vi "Generate Bursted Script.vi"(0 "PAEN Config":T1={"PAEN Mode"=enum."Dynamic", "PA Enable Trigger Export Terminal"="PFI0", "PA Enable Trigger Mode"=23001, "Command Enable Time (s)"=0.0, "Command Disable Time (s)"=0.0} {"PA Enable Trigger Mode" items=["Pulse"=23000, "Toggle"=23001]; "Command Disable Time (s)" format="%#_6p"; "Command Enable Time (s)" format="%#_6p"}, 5 "Waveform Timing Configuration":T4 {"Post-Burst Time (s)" format="%#_6p"; "Pre-Burst Time (s)" format="%#_6p"; "Duty Cycle (%)" min=1.0 max=100.0 step=1.0 format="%#_2d%%"}, 7 "Waveform":T3 {"Runtime Scaling" format="%#_6p"; "Sample Rate" format="%#_6p"; "Burst Length (s)" format="%#_6p"; "PAPR (dB)" format="%.2f"; "Signal Bandwidth (Hz)" format="%#_6p"}, 11 "error in (no error)":errorcluster) -> (4 "Script":string, 6 "Generation Period (s)":dbl, 15 "error out":errorcluster)   [LabVIEW 2019, in "SG.lvlib"]
doc: "Creates the generation script used for bursted generation."
uses:
  SG.lvlib
  Typedefs/Waveform Timing Configuration.ctl
  <instrlib>/niRFSG/niRFSG.llb/niRFSG Exported Signal Destinations.ctl
  Common/Waveform.ctl
  Typedefs/PAEN Configuration.ctl
  <vilib>/Utility/error.llb/Error Cluster From Error Code.vi
  <vilib>/ErrorRing/Error Ring.xnode
  Common/Common.lvlib
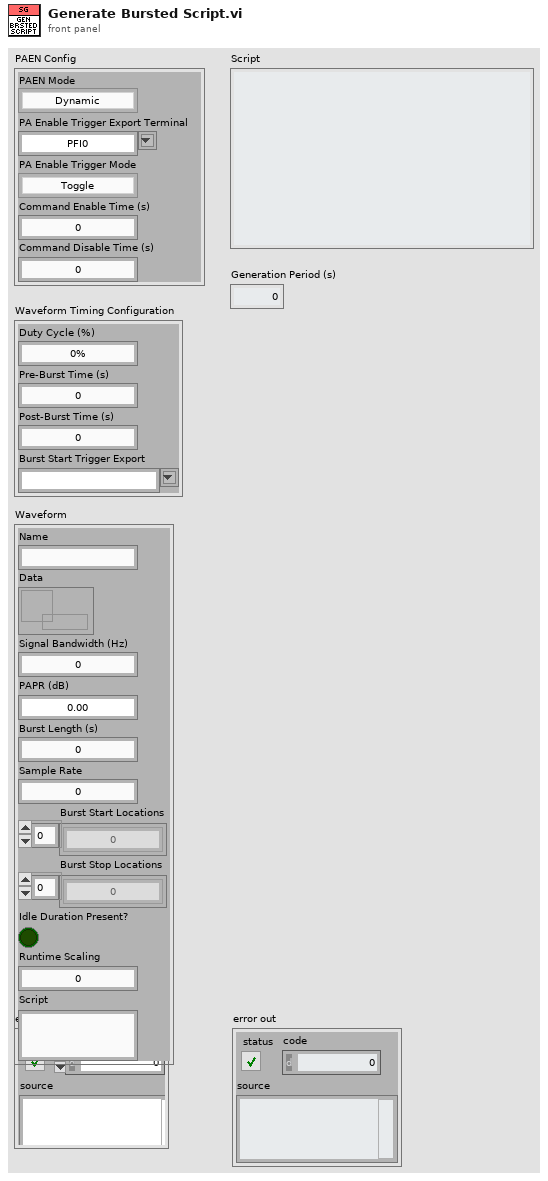
[diagram p1: front panel]
types:
  T1 = typedef "SG.lvlib/PAEN Configuration.ctl" = cluster{"PAEN Mode":enum16{"Disabled", "Static", "Dynamic"}, "PA Enable Trigger Export Terminal":T2, "PA Enable Trigger Mode":i32, "Command Enable Time (s)":dbl, "Command Disable Time (s)":dbl}
  T2 = typedef "niRFSG Exported Signal Destinations.ctl" = string
  T3 = typedef "Common.lvlib/Waveform.ctl" = cluster{"Name":string, "Data":refnum<data-value>, "Signal Bandwidth (Hz)":dbl, "PAPR (dB)":dbl, "Burst Length (s)":dbl, "Sample Rate":dbl, "Burst Start Locations":i32[], "Burst Stop Locations":i32[], "Idle Duration Present?":bool, "Runtime Scaling":dbl, "Script":string}
  T4 = typedef "SG.lvlib/Waveform Timing Configuration.ctl" = cluster{"Duty Cycle (%)":dbl, "Pre-Burst Time (s)":dbl, "Post-Burst Time (s)":dbl, "Burst Start Trigger Export":T2}
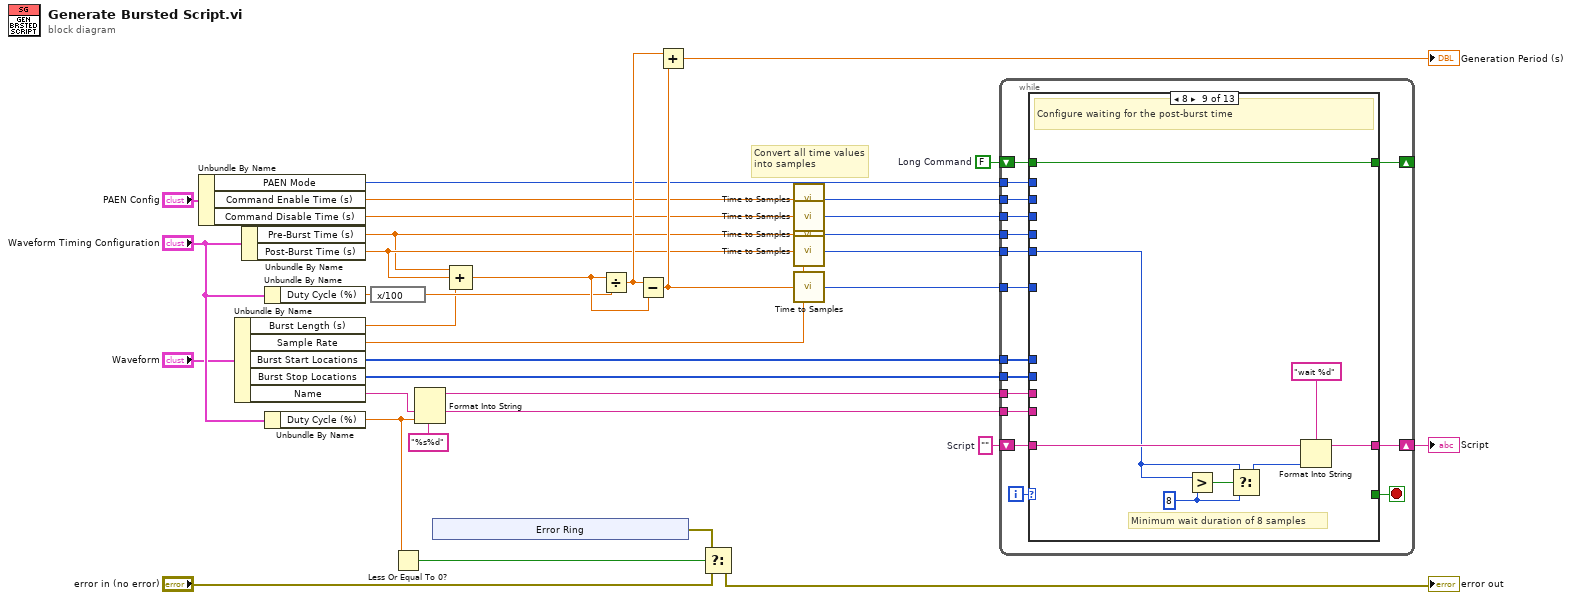
[diagram p0: block diagram]
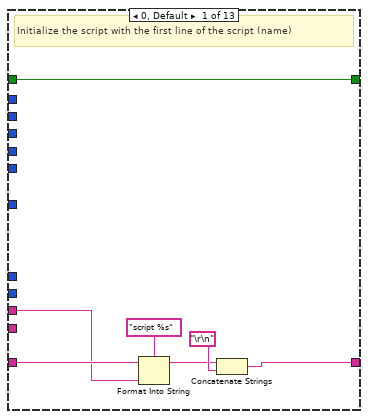
[diagram p2: hidden frame]
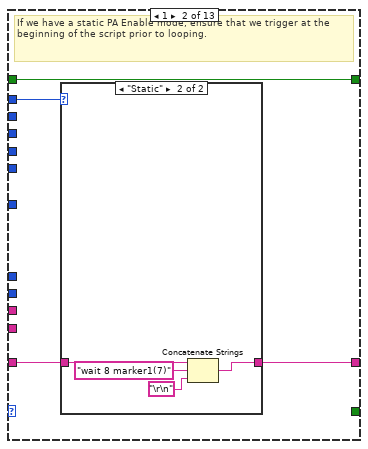
[diagram p3: hidden frame]
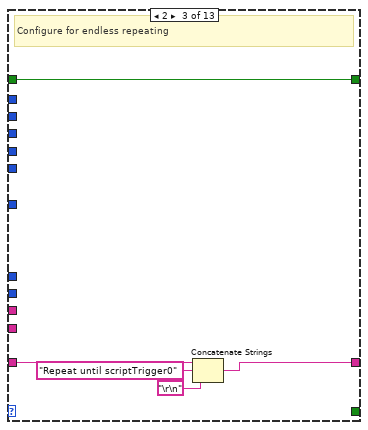
[diagram p5: hidden frame]
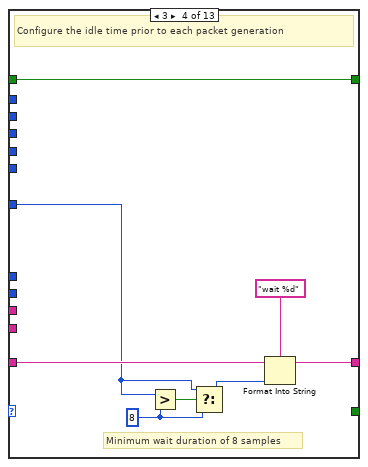
[diagram p6: hidden frame]
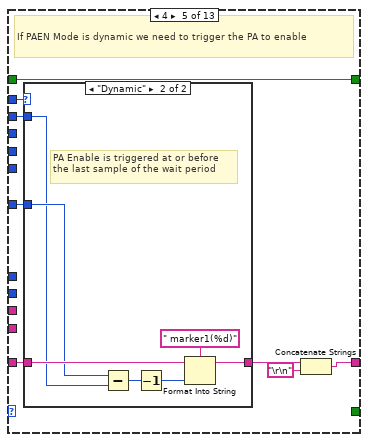
[diagram p7: hidden frame]
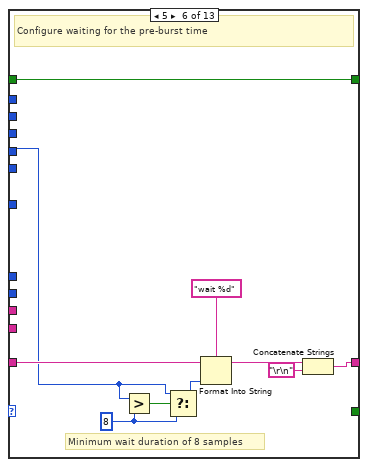
[diagram p9: hidden frame]
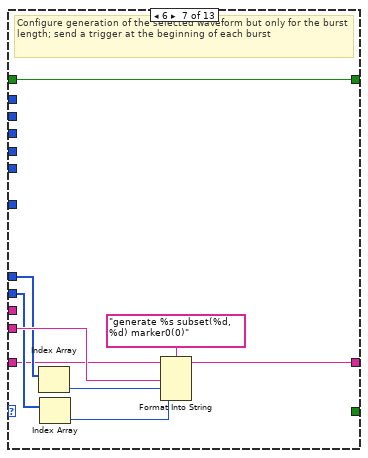
[diagram p10: hidden frame]
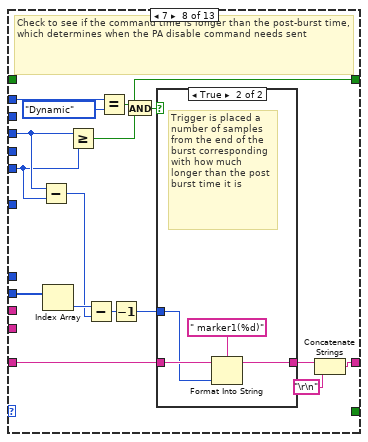
[diagram p11: hidden frame]
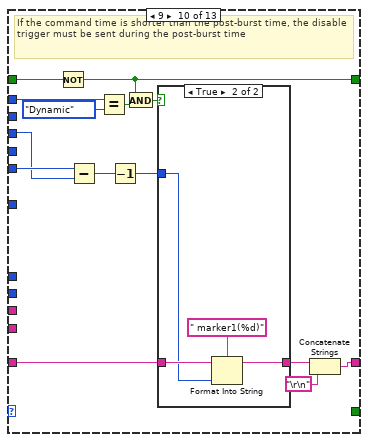
[diagram p13: hidden frame]
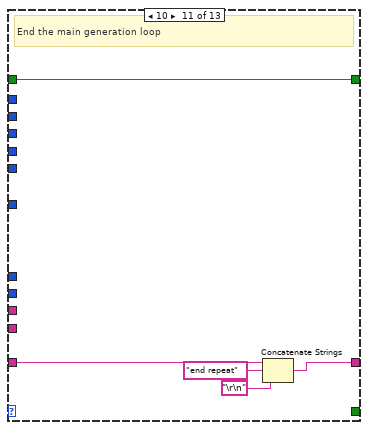
[diagram p15: hidden frame]
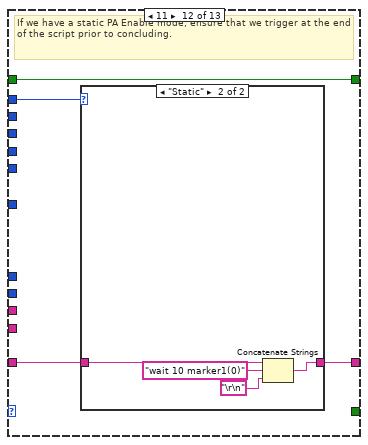
[diagram p16: hidden frame]
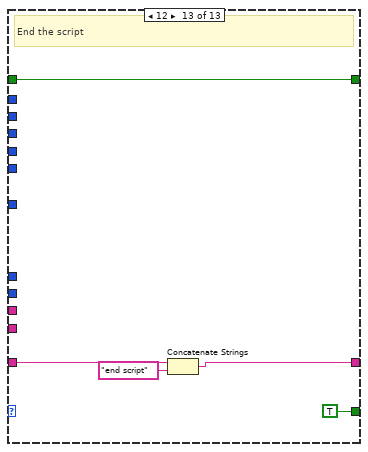
[diagram p18: hidden frame]
diagram:
  w30 = FALSE  # Long Command
  w25 = ""  # Script
  # "Convert all time values into samples"
  n1 = Unbundle By Name("PAEN Config") -> ("PAEN Mode"=w26:enum16{"Disabled", "Static", "Dynamic"}, "Command Enable Time (s)"=w9:dbl, "Command Disable Time (s)"=w10:dbl)
  n2 = Unbundle By Name("Waveform") -> ("Burst Length (s)"=w13:dbl, "Sample Rate"=w18:dbl, "Burst Start Locations"=w28:i32[], "Burst Stop Locations"=w29:i32[], "Name"=w27:string)
  n3 = Unbundle By Name("Waveform Timing Configuration") -> ("Pre-Burst Time (s)"=w11:dbl, "Post-Burst Time (s)"=w12:dbl)
  n4 = Unbundle By Name("Waveform Timing Configuration") -> ("Duty Cycle (%)"=w15:dbl)
  n5 = Unbundle By Name("Waveform Timing Configuration") -> ("Duty Cycle (%)"=w32:dbl)
  n6 = expression code="x/100"(w15) -> (w16:dbl)
  n7 = Less Or Equal To 0?(x=w32) -> (x <= 0?=w6:bool)
  n8 = Format Into String(format string="%s%d", w27, w32) -> (resulting string=w24:string)  [unwired: 2 in, 1 out]
  n9 = xnode "Error Ring"() -> ("error out"=w1:errorcluster)
  n10 = Compound Arithmetic op=ADD(w11, w12, w13) -> (w17:dbl)
  n11 = Divide(x=w17, y=w16) -> (x/y=w33:dbl)
  n12 = Subtract(x=w33, y=w17) -> (x-y=w34:dbl)
  n13 = Add(x=w33, y=w34) -> (x+y=→"Generation Period (s)":dbl)
  n14 = Select(t=w1, s=w6, f="error in (no error)") -> (s? t:f=→"error out":errorcluster)
  n15 = call "Time to Samples.vi"("Time"=w9, "Sample Rate"=w18) -> ("Samples"=w19:u32)  [unwired: 13 in]
  n16 = call "Time to Samples.vi"("Time"=w10, "Sample Rate"=w18) -> ("Samples"=w20:u32)  [unwired: 13 in]
  n17 = call "Time to Samples.vi"("Time"=w11, "Sample Rate"=w18) -> ("Samples"=w21:u32)  [unwired: 13 in]
  n18 = call "Time to Samples.vi"("Time"=w12, "Sample Rate"=w18) -> ("Samples"=w22:u32)  [unwired: 13 in]
  n19 = call "Time to Samples.vi"("Time"=w34, "Sample Rate"=w18) -> ("Samples"=w23:u32)  [unwired: 13 in]
  n20 = while {
    tunnel: w19 -> [w43]
    tunnel: w20 -> [w38]
    tunnel: w21 -> [w45]
    tunnel: w22 -> [w39]
    tunnel: w23 -> [w44]
    tunnel: w24 -> [w48]
    shift-right: [w47] -> w31
    shift-left: w25 -> [w49]
    tunnel: w26 -> [w46]
    tunnel: w27 -> [w42]
    tunnel: w28 -> [w41]
    tunnel: w29 -> [w40]
    shift-right: [w37] -> _
    shift-left: w30 -> [w36]
    i -> [w50]
    stop <- w35 stop-if-true
    n21 = case shown="8" w50 {
      tunnel: w49 -> [w57 w60 w71 w79 w87 w105 w109 w127 w143 w154 w165 w171 w180]
      tunnel: w48 -> [w55 _ _ _ _ _ _ _ _ _ _ _ _]
      tunnel: [w52 w59 w70 w77 w81 w101 w113 w120 w141 w151 w167 w170 w179] -> w47
      tunnel: w46 -> [_ w61 _ _ w86 _ _ w130 _ w157 _ w168 _]
      tunnel: w45 -> [_ _ _ _ _ w96 _ _ _ _ _ _ _]
      tunnel: w44 -> [_ _ _ w75 w84 _ _ _ _ _ _ _ _]
      tunnel: w43 -> [_ _ _ _ w85 _ _ _ _ _ _ _ _]
      tunnel: w42 -> [_ _ _ _ _ _ w112 _ _ _ _ _ _]
      tunnel: w41 -> [_ _ _ _ _ _ w111 _ _ _ _ _ _]
      tunnel: w40 -> [_ _ _ _ _ _ w110 w124 _ _ _ _ _]
      tunnel: w39 -> [_ _ _ _ _ _ _ w117 w136 w148 _ _ _]
      tunnel: w38 -> [_ _ _ _ _ _ _ w118 _ w147 _ _ _]
      tunnel: [w51 w58 w67 w76 w80 w100 w106 w115 w140 w144 w166 w169 w181] -> w37
      tunnel: w36 -> [w51 w58 w67 w76 w80 w100 w106 _ w140 w149 w166 w169 w181]
      tunnel: [_ _ _ _ _ _ _ _ _ _ _ _ TRUE] -> w35
      frame 0, Default {
        # "Initialize the script with the first line of the script (name)"
        n22 = Format Into String(format string="script %s", initial string=w57, w55) -> (resulting string=w53:string)  [unwired: 1 in, 1 out]
        n23 = Concatenate Strings(w53, "\r\n") -> (w52:string)
      }
      frame 1 {
        # "If we have a static PA Enable mode, ensure that we trigger at the beginning of the script prior to looping."
        n24 = case shown="\"Static\"" w61 {
          tunnel: w60 -> [w62 w66]
          tunnel: [w62 w65] -> w59
          frame Default {
          }
          frame "Static" {
            n25 = Concatenate Strings(w66, "wait 8 marker1(7)", "\r\n") -> (w65:string)
          }
        }
      }
      frame 2 {
        # "Configure for endless repeating"
        n26 = Concatenate Strings(w71, "Repeat until scriptTrigger0" ("string"), "\r\n" ("string")) -> (w70:string)
      }
      frame 3 {
        w73 = u32 8 ("y")
        # "Minimum wait duration of 8 samples"
        # "Configure the idle time prior to each packet generation"
        n27 = Greater?(x=w75, y=w73) -> (0:w74:bool)
        n28 = Select(t=w75, s=w74, f=w73) -> (s? t:f=w72:u32)
        n29 = Format Into String(format string="wait %d", initial string=w79, w72) -> (resulting string=w77:string)  [unwired: 1 in, 1 out]
      }
      frame 4 {
        # "If PAEN Mode is dynamic we need to trigger the PA to enable"
        n30 = case shown="\"Dynamic\"" w86 {
          tunnel: w87 -> [w88 w95]
          tunnel: [w88 w93] -> w82
          tunnel: w85 -> [_ w91]
          tunnel: w84 -> [_ w92]
          frame Default {
          }
          frame "Dynamic" {
            # "PA Enable is triggered at or before the last sample of the wait period"
            n31 = Subtract(x=w92, y=w91) -> (x-y=w90:u32)
            n32 = Decrement(x=w90) -> (x-1=w89:u32)
            n33 = Format Into String(format string=" marker1(%d)", initial string=w95, w89) -> (resulting string=w93:string)  [unwired: 1 in, 1 out]
          }
        }
        n34 = Concatenate Strings(w82, "\r\n" ("string")) -> (w81:string)
      }
      frame 5 {
        w98 = u32 8 ("y")
        # "Minimum wait duration of 8 samples"
        # "Configure waiting for the pre-burst time"
        n35 = Greater?(x=w96, y=w98) -> (0:w99:bool)
        n36 = Select(t=w96, s=w99, f=w98) -> (s? t:f=w97:u32)
        n37 = Format Into String(format string="wait %d", initial string=w105, w97) -> (resulting string=w102:string)  [unwired: 1 in, 1 out]
        n38 = Concatenate Strings(w102, "\r\n" ("string")) -> (w101:string)
      }
      frame 6 {
        # "Configure generation of the selected waveform but only for the burst length; send a trigger at the beginning of each burst"
        n39 = Index Array(array=w111) -> (element=w108:i32)  [unwired: 1 in]
        n40 = Index Array(array=w110) -> (element=w107:i32)  [unwired: 1 in]
        n41 = Format Into String(format string="generate %s subset(%d, %d) marker0(0)", initial string=w109, w112, w108, w107) -> (resulting string=w113:string)  [unwired: 1 in, 1 out]
      }
      frame 7 {
        # "Check to see if the command time is longer than the post-burst time, which determines when the PA disable command needs sent"
        n42 = Subtract(x=w118, y=w117) -> (x-y=w122:u32)
        n43 = Index Array(array=w124) -> (element=w123:i32)  [unwired: 1 in]
        n44 = Greater Or Equal?(x=w118, y=w117) -> (x >= y?=w115:bool)
        n45 = Subtract(x=w123, y=w122) -> (x-y=w121:u32)
        n46 = Equal?(x=w130, y=enum16{"Disabled", "Static", "Dynamic"}."Dynamic") -> (x = y?=w128:bool)
        n47 = Decrement(x=w121) -> (x-1=w116:u32)
        n48 = And(x=w128, y=w115) -> (x .and. y?=w125:bool)
        n49 = case shown="True" w125 {
          tunnel: w127 -> [w131 w135]
          tunnel: [w131 w134] -> w126
          tunnel: w116 -> [_ w132]
          frame False {
          }
          frame True {
            # "Trigger is placed a number of samples from the end of the burst corresponding with how much longer than the post burst time it is"
            n50 = Format Into String(format string=" marker1(%d)", initial string=w135, w132) -> (resulting string=w134:string)  [unwired: 1 in, 1 out]
          }
        }
        n51 = Concatenate Strings(w126, "\r\n" ("string")) -> (w120:string)
      }
      frame 8 {
        w138 = u32 8 ("y")
        # "Minimum wait duration of 8 samples"
        # "Configure waiting for the post-burst time"
        n52 = Greater?(x=w136, y=w138) -> (0:w139:bool)
        n53 = Select(t=w136, s=w139, f=w138) -> (s? t:f=w137:u32)
        n54 = Format Into String(format string="wait %d", initial string=w143, w137) -> (resulting string=w141:string)  [unwired: 1 in, 1 out]
      }
      frame 9 {
        # "If the command time is shorter than the post-burst time, the disable trigger must be sent during the post-burst time"
        n55 = Not(x=w149) -> (.not. x?=w144:bool)
        n56 = Subtract(x=w148, y=w147) -> (x-y=w146:u32)
        n57 = Equal?(x=w157, y=enum16{"Disabled", "Static", "Dynamic"}."Dynamic") -> (x = y?=w155:bool)
        n58 = Decrement(x=w146) -> (x-1=w145:u32)
        n59 = And(x=w144, y=w155) -> (x .and. y?=w152:bool)
        n60 = case shown="True" w152 {
          tunnel: w154 -> [w158 w162]
          tunnel: [w158 w161] -> w153
          tunnel: w145 -> [_ w159]
          frame False {
          }
          frame True {
            n61 = Format Into String(format string=" marker1(%d)", initial string=w162, w159) -> (resulting string=w161:string)  [unwired: 1 in, 1 out]
          }
        }
        n62 = Concatenate Strings(w153, "\r\n" ("string")) -> (w151:string)
      }
      frame 10 {
        # "End the main generation loop"
        n63 = Concatenate Strings(w165, "end repeat" ("format string"), "\r\n" ("string")) -> (w167:string)
      }
      frame 11 {
        # "If we have a static PA Enable mode, ensure that we trigger at the end of the script prior to concluding."
        n64 = case shown="\"Static\"" w168 {
          tunnel: w171 -> [w172 w174]
          tunnel: [w172 w175] -> w170
          frame Default {
          }
          frame "Static" {
            n65 = Concatenate Strings(w174, "wait 10 marker1(0)" ("format string"), "\r\n" ("string")) -> (w175:string)
          }
        }
      }
      frame 12 {
        # "End the script"
        n66 = Concatenate Strings(w180, "end script" ("string")) -> (w179:string)
      }
    }
  }
  "Script" <- w31
